vi "HEWH Inlet Outlet Temperature Average.vi"(0 "Remove 15 Seconds Input":T2 {"Hot Water Total (Gal)" format="%#.6f"; "Software Elapsed Time (s)" format="%#.6f"; "Cold Water Total (Gal)" format="%#.6f"}, 1 "Test Type":T1, 11 "error in (no error)":errorcluster) -> (4 "Remove 15 Seconds Output":T2 {"Hot Water Total (Gal)" format="%#.6f"; "Software Elapsed Time (s)" format="%#.6f"; "Cold Water Total (Gal)" format="%#.6f"}, 14 "Time_15s":dbl, 15 "error out":errorcluster)   [LabVIEW 2023]
uses:
  Type Definitions/HEWH Remove 15 Seconds.ctl
  Type Definitions/HEWH Test Type.ctl
panel:
  out "Array":dbl[][](array[numeric])
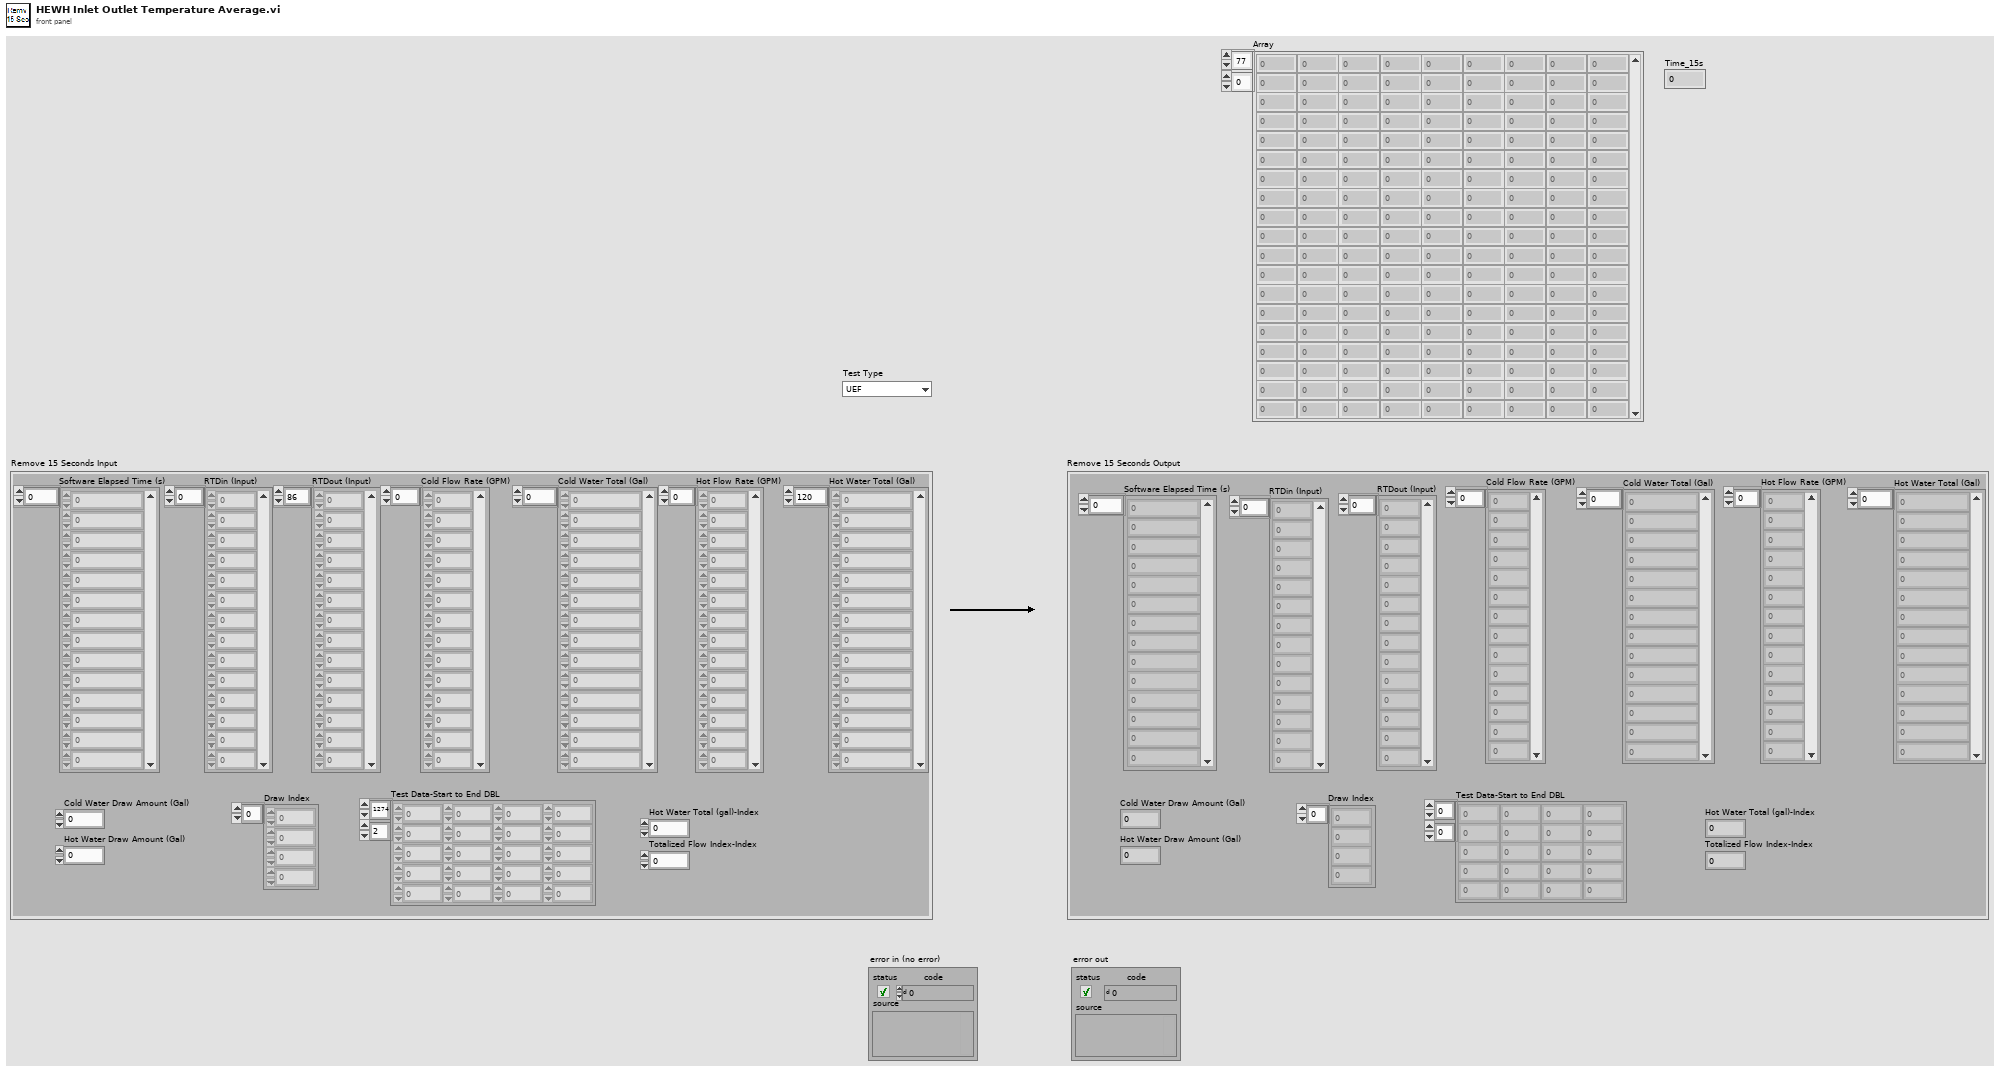
[diagram p1: front panel]
types:
  T1 = typedef "HEWH Test Type.ctl" = enum16{"UEF", "FHD"}
  T2 = typedef "HEWH Remove 15 Seconds.ctl" = cluster{"Cold Water Total (Gal)":dbl[], "Software Elapsed Time (s)":dbl[], "RTDin (Input)":dbl[], "RTDout (Input)":dbl[], "Cold Flow Rate (GPM)":dbl[], "Hot Flow Rate (GPM)":dbl[], "Hot Water Total (Gal)":dbl[], "Cold Water Draw Amount (Gal)":dbl, "Hot Water Draw Amount (Gal)":dbl, "Draw Index":i32[], "Test Data-Start to End DBL":dbl[][], "Hot Water Total (gal)-Index":i32, "Totalized Flow Index-Index":i32}
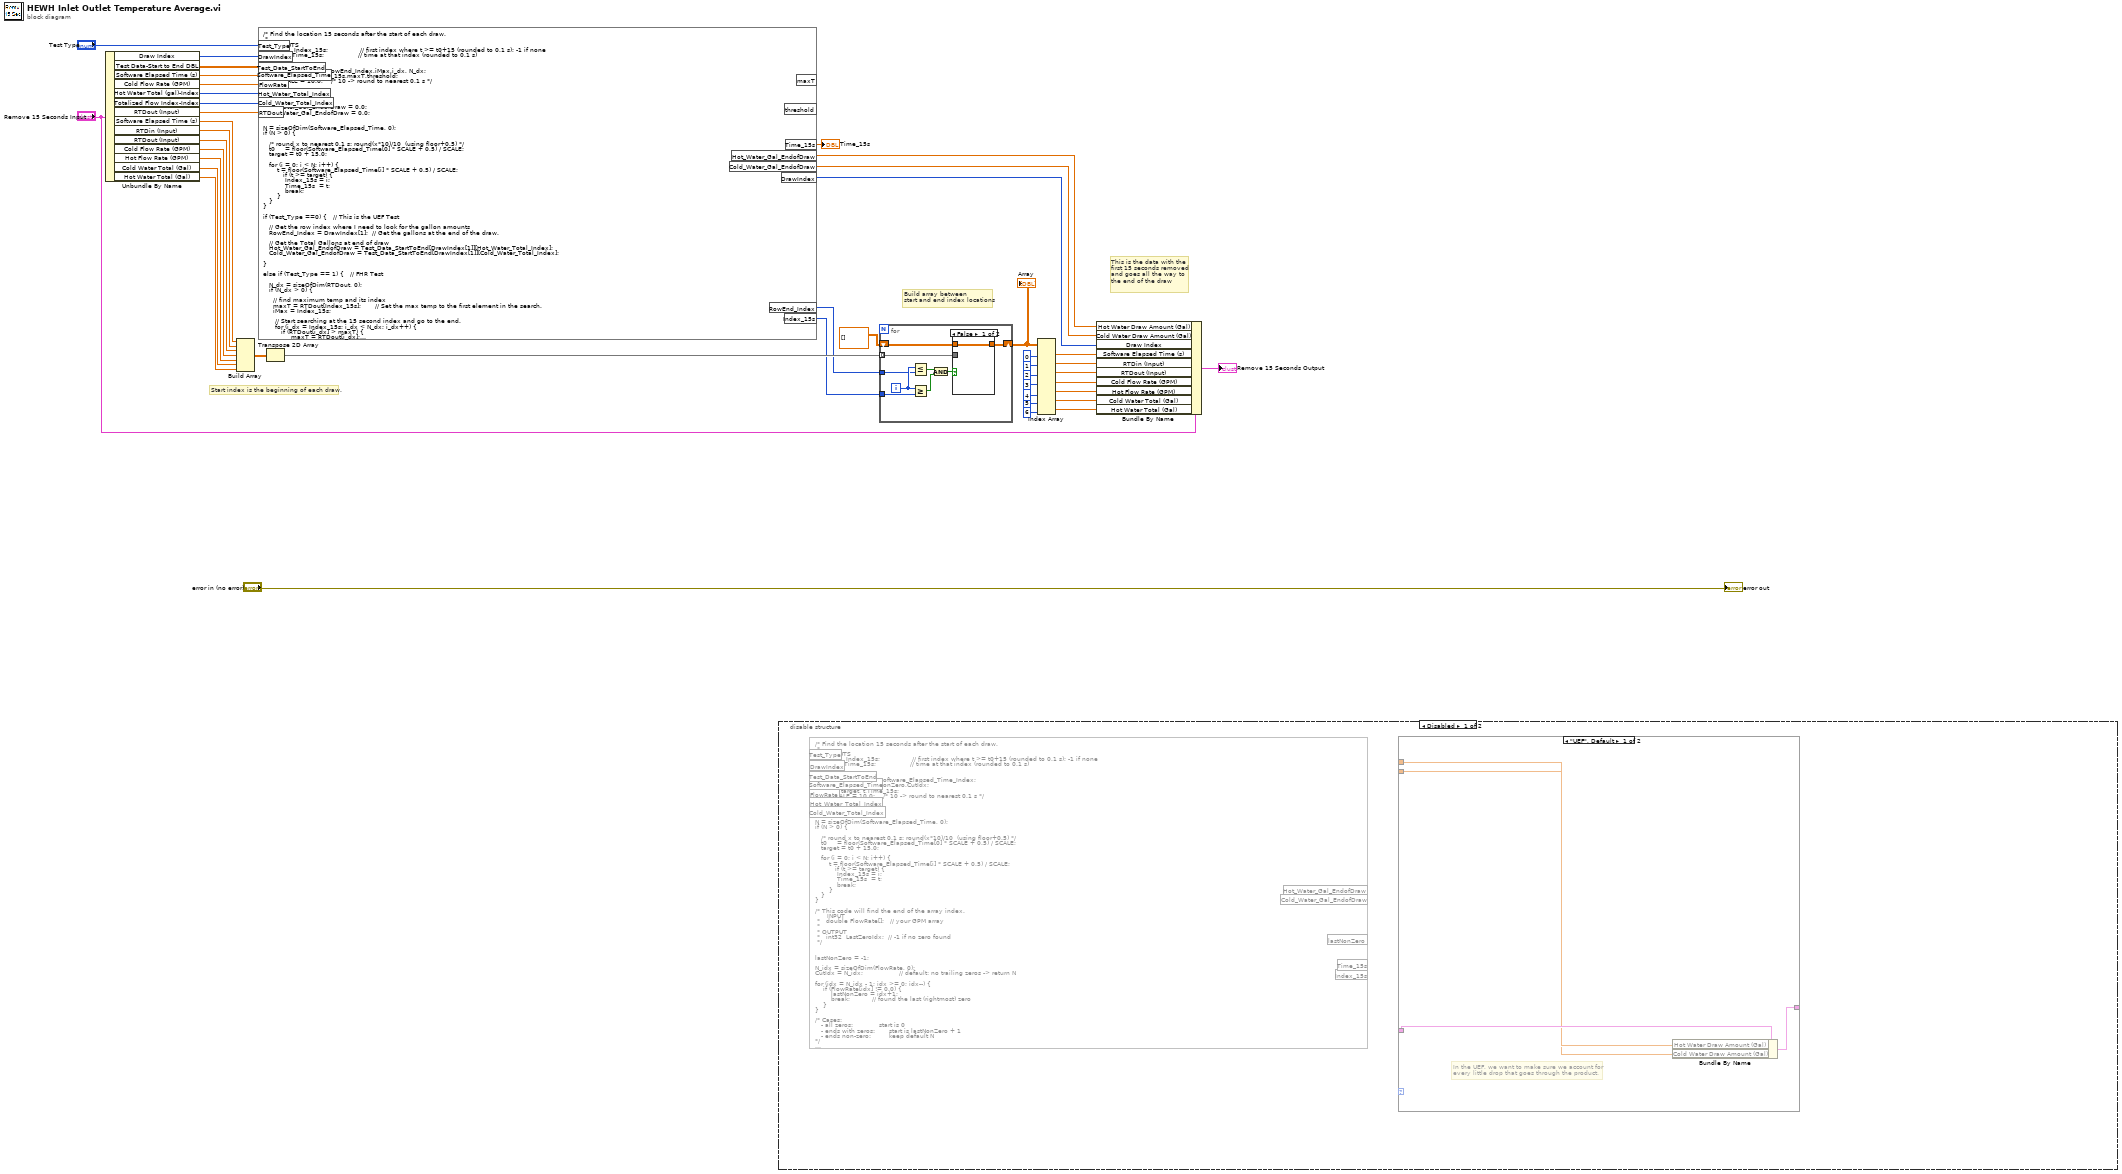
[diagram p0: block diagram]
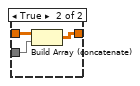
[diagram p2: hidden frame]
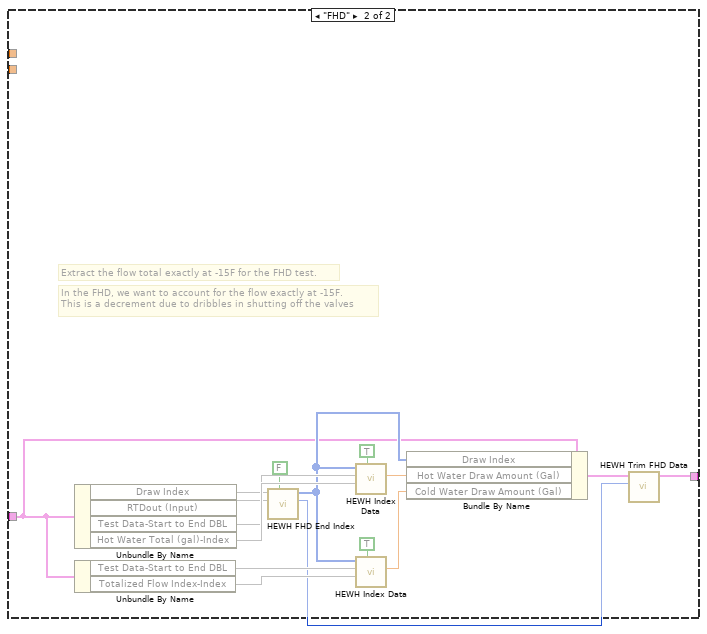
[diagram p3: hidden frame]
diagram:
  # "Start index is the beginning of each draw."
  # "Build array between\nstart and end index locations"
  # "This is the data with the\nfirst 15 seconds removed\nand goes all the way to\nthe end of the draw"
  n1 = Unbundle By Name("Remove 15 Seconds Input") -> ("Draw Index"=w23:i32[], "Test Data-Start to End DBL"=w22:dbl[][], "Software Elapsed Time (s)"=w32:dbl[], "Cold Flow Rate (GPM)"=w33:dbl[], "Hot Water Total (gal)-Index"=w20:i32, "Totalized Flow Index-Index"=w19:i32, "RTDout (Input)"=w18:dbl[], "Software Elapsed Time (s)"=w35:dbl[], "RTDin (Input)"=w40:dbl[], "RTDout (Input)"=w39:dbl[], "Cold Flow Rate (GPM)"=w38:dbl[], "Hot Flow Rate (GPM)"=w37:dbl[], "Cold Water Total (Gal)"=w36:dbl[], "Hot Water Total (Gal)"=w34:dbl[])
  n2 = Build Array(w35, w40, w39, w38, w37, w36, w34) -> (w41:dbl[][])
  n3 = formula code="/* Find the location 15 seconds after the start of each draw. \n *\n * OUTPUTS\n *   int32  Index_15s;                // first index where t >= t0+15 (rounded to 0.1 s); -1 if none\n *   float  Time_15s;                 // time at that index (rounded to 0.1 s)\n */\n\nint32 i, N,Index_15s,RowEnd_Index,iMax,i_dx, N_dx;\nfloat t0, target, t,Time_15s,maxT,threshold;\nfloat SCALE = 10.0;    /* 10 -> round to nearest 0.1 s */\n\nIndex_15s = -1;\nTime_15s  = 0.0;\nRowEnd_Index = -1;\nHot_Water_Gal_EndofDraw = 0.0;\nCold_Water_Gal_EndofDraw = 0.0;\n\n\nN = sizeOfDim(Software_Elapsed_Time, 0);\nif (N > 0) {\n\n   /* round x to nearest 0.1 s: round(x*10)/10  (using floor+0.5) */\n   t0     = floor(Software_Elapsed_Time[0] * SCALE + 0.5) / SCALE;\n   target = t0 + 15.0;\n\n   for (i = 0; i < N; i++) {\n       t = floor(Software_Elapsed_Time[i] * SCALE + 0.5) / SCALE;\n          if (t >= target) {\n           Index_15s = i;\n           Time_15s  = t;\n           break;\n       }\n   }\n}\n\nif (Test_Type ==0) {   // This is the UEF Test\n\n   // Get the row index where I need to look for the gallon amounts\n   RowEnd_Index = DrawIndex[1];  // Get the gallons at the end of the draw.\n\n   // Get the Total Gallons at end of draw\n   Hot_Water_Gal_EndofDraw = Test_Data_StartToEnd[DrawIndex[1]][Hot_Water_Total_Index];\n   Cold_Water_Gal_EndofDraw = Test_Data_StartToEnd[DrawIndex[1]][Cold_Water_Total_Index];\n\n}\n\nelse if (Test_Type == 1) {   // FHR Test\n\n   N_dx = sizeOfDim(RTDout, 0);\n   if (N_dx > 0) {\n     \n     // find maximum temp and its index\n     maxT = RTDout[Index_15s];       // Set the max temp to the first element in the search.\n     iMax = Index_15s;\n\n      // Start searching at the 15 second index and go to the end.\n      for (i_dx = Index_15s; i_dx < N_dx; i_dx++) {\n         if (RTDout[i_dx] > maxT) { \n              maxT = RTDout[i_dx];\n              iMax = i_dx;\n         }\n      }\n\n      // threshold at max - 15°F\n      threshold = maxT - 15.0;\n      \n      // reset for this branch\n      RowEnd_Index = -1;\n\n      // *** scan forward from the maximum index ***\n      for (i_dx = iMax; i_dx <= N_dx; i_dx++) {\n          if (RTDout[i_dx] <= threshold) {\n            RowEnd_Index = i_dx;   // first point = (maxT - 15)\n            break;\n         }\n      }\n\n       // Get the absolute array position for Draw Index (this is the end position)\n       DrawIndex[1] = DrawIndex[0] + RowEnd_Index;   /* absolute end-of-draw position */ \n\n      // grab gallons at that index if found\n      if (RowEnd_Index >= 0 && RowEnd_Index < sizeOfDim(Test_Data_StartToEnd, 0)) {\n         Hot_Water_Gal_EndofDraw  = Test_Data_StartToEnd[DrawIndex[1]][Hot_Water_Total_Index];;\n         Cold_Water_Gal_EndofDraw = Test_Data_StartToEnd[DrawIndex[1]][Cold_Water_Total_Index];\n      }\n   }\n}"("FlowRate"=w33, "Software_Elapsed_Time"=w32, "DrawIndex"=w23, "Test_Data_StartToEnd"=w22, "Test_Type"="Test Type", "Hot_Water_Total_Index"=w20, "Cold_Water_Total_Index"=w19, "RTDout"=w18) -> ("RowEnd_Index"=w13:i32, "Index_15s"=w14:i32, "Time_15s"=→"Time_15s":dbl, "Hot_Water_Gal_EndofDraw"=w4:dbl, "Cold_Water_Gal_EndofDraw"=w3:dbl, "DrawIndex"=w5:i32[])  [unwired: 2 out]
  n4 = Transpose 2D Array(2D array=w41) -> (transposed array=w17:dbl[][])
  n5 = disable-structure shown="Disabled" {
    frame Disabled {
      n6 = formula code="/* Find the location 15 seconds after the start of each draw. \n *\n * OUTPUTS\n *   int32  Index_15s;                // first index where t >= t0+15 (rounded to 0.1 s); -1 if none\n *   float  Time_15s;                 // time at that index (rounded to 0.1 s)\n */\n\nint32 i, N,Index_15s,Software_Elapsed_Time_Index;\nint32 idx, N_idx, lastNonZero,CutIdx;\nfloat t0, target, t,Time_15s;\nfloat SCALE = 10.0;    /* 10 -> round to nearest 0.1 s */\n\nIndex_15s = -1;\nTime_15s  = 0.0;\n\nN = sizeOfDim(Software_Elapsed_Time, 0);\nif (N > 0) {\n\n   /* round x to nearest 0.1 s: round(x*10)/10  (using floor+0.5) */\n   t0     = floor(Software_Elapsed_Time[0] * SCALE + 0.5) / SCALE;\n   target = t0 + 15.0;\n\n   for (i = 0; i < N; i++) {\n       t = floor(Software_Elapsed_Time[i] * SCALE + 0.5) / SCALE;\n          if (t >= target) {\n           Index_15s = i;\n           Time_15s  = t;\n           break;\n       }\n   }\n}\n\n/* This code will find the end of the array index.  \n      INPUT\n *   double FlowRate[];   // your GPM array\n *\n * OUTPUT\n *   int32  LastZeroIdx;  // -1 if no zero found\n */\n\n\nlastNonZero = -1;\n\nN_idx = sizeOfDim(FlowRate, 0);\nCutIdx = N_idx;                  // default: no trailing zeros -> return N\n\nfor (idx = N_idx - 1; idx >= 0; idx--) {\n    if (FlowRate[idx] != 0.0) {\n        lastNonZero = idx+1;\n        break;           // found the last (rightmost) zero\n    }\n}\n\n/* Cases:\n   - all zeros:             start is 0\n   - ends with zeros:       start is lastNonZero + 1\n   - ends non-zero:         keep default N\n*/\n\nif (lastNonZero == -1) {\n    CutIdx = 0;                 // e.g., [0,0,0] -> 0\n} \nelse if (lastNonZero < N_idx - 1) {\n    CutIdx = lastNonZero+1;   // e.g., [20,0,0,0] -> 1\n}\n/* else leave CutIdx = N (e.g., [1,2,3] -> 3) */\n\n// This section of code finds the hot and cold water totalized gallons\n\nif (Test_Type ==0) {   // This is the UEF Test\n\n// Get the row index where I need to look for the gallon amounts\nSoftware_Elapsed_Time_Index = DrawIndex[1];\n\n// Get the Total Gallons\nHot_Water_Gal_EndofDraw = Test_Data_StartToEnd[Software_Elapsed_Time_Index][Hot_Water_Total_Index];\nCold_Water_Gal_EndofDraw = Test_Data_StartToEnd[Software_Elapsed_Time_Index][Cold_Water_Total_Index];\n\n}\n\n// In this section, I need to look for -15F decrement exactly and get that location.\n// So, look at the RTDout, find the maximum temperature in the draw, then subtract 15 degrees, then move \n// your index backward until you get a 15 degree decrement, this is your new stop index. This is index location is\n// your new \"lastNonZero\" index location. then go ahead and grab the \"Hot_Water_Gal_EndofDraw\" and\n// \"Cold_Water_Gal_EndofDraw\""() -> ()  [unwired: 7 in, 5 out]
      n7 = case shown="\"UEF\", Default" {
        selector: _ -> [_ _]
        tunnel: _ -> [w45 w47]
        tunnel: [w46 w49] -> _
        tunnel: _ -> [w44 _]
        tunnel: _ -> [w43 _]
        frame "UEF", Default {
          # "In the UEF, we want to make sure we account for\nevery little drop that goes through the product."
          n8 = Bundle By Name(cluster=w45, "Hot Water Draw Amount (Gal)"=w44, "Cold Water Draw Amount (Gal)"=w43) -> (w46:cluster{})
        }
        frame "FHD" {
          # "In the FHD, we want to account for the flow exactly at -15F.\nThis is a decrement due to dribbles in shutting off the valves"
          # "Extract the flow total exactly at -15F for the FHD test."
          n9 = Unbundle By Name(w47) -> ("Draw Index"=w57, "RTDout (Input)"=w56, "Test Data-Start to End DBL"=w55, "Hot Water Total (gal)-Index"=w61)
          n10 = Unbundle By Name(w47) -> ("Test Data-Start to End DBL"=w59, "Totalized Flow Index-Index"=w60)
          n11 = call "HEWH FHD End Index.vi"("Fixed Search?"=FALSE, "RTDout"=w56, "Draw Index"=w57) -> ("Decrement Amount"=w51:i32, "Updated FHD End Index"=w54:i32[])  [unwired: 6 in, 1 out]
          n12 = call "HEWH Index Data.vi"("Basic Index?"=TRUE, "Data Index Location"=w61, "Test Data-Start to End DBL"=w55, "Draw Index"=w54) -> ("Basic Index Output"=w53:dbl)  [unwired: 5 in, 2 out]
          n13 = call "HEWH Index Data.vi"("Basic Index?"=TRUE, "Data Index Location"=w60, "Test Data-Start to End DBL"=w59, "Draw Index"=w54) -> ("Basic Index Output"=w52:dbl)  [unwired: 5 in, 2 out]
          n14 = Bundle By Name(cluster=w47, "Draw Index"=w54, "Hot Water Draw Amount (Gal)"=w53, "Cold Water Draw Amount (Gal)"=w52) -> (w50:cluster{})
          n15 = call "HEWH Trim FHD Data.vi"("Decrement Amount"=w51, "Remove 15 Seconds Input in"=w50) -> ("Remove 15 Seconds Input out"=w49:T2)  [unwired: 8 in, 1 out]
        }
      }
    }
    frame Enabled {
    }
  }
  n16 = for {
    tunnel: w17 -> [w71] mode=indexing
    shift-right: [w69] -> w15
    shift-left: dbl[][] [] -> [w70]
    tunnel: w13 -> [w66]
    tunnel: w14 -> [w68]
    i -> [w67]
    n17 = Less Or Equal?(x=w67, y=w66) -> (x <= y?=w65:bool)
    n18 = Greater Or Equal?(x=w67, y=w68) -> (x >= y?=w64:bool)
    n19 = And(x=w65, y=w64) -> (x .and. y?=w63:bool)
    n20 = case shown="False" w63 {
      tunnel: w71 -> [_ w75]
      tunnel: w70 -> [w72 w74]
      tunnel: [w72 w73] -> w69
      frame False {
      }
      frame True {
        n21 = Build Array (concatenate)(w74, w75) -> (w73:dbl[][])
      }
    }
  }
  "Array" <- w15
  n22 = Index Array(array=w15, index (col) #1=0 ("disabled index (col)"), index (col) #2=1 ("index (col)"), index (col) #3=2 ("index (col)"), index (col) #4=3 ("index (col)"), index (col) #5=4 ("index (col)"), index (col) #6=5 ("index (col)"), index (col) #7=6 ("index (col)")) -> (element #1=w12:dbl[], element #2=w11:dbl[], element #3=w10:dbl[], element #4=w9:dbl[], element #5=w8:dbl[], element #6=w7:dbl[], element #7=w6:dbl[])  [unwired: 7 in]
  n23 = Bundle By Name(cluster="Remove 15 Seconds Input", "Hot Water Draw Amount (Gal)"=w4, "Cold Water Draw Amount (Gal)"=w3, "Draw Index"=w5, "Software Elapsed Time (s)"=w12, "RTDin (Input)"=w11, "RTDout (Input)"=w10, "Cold Flow Rate (GPM)"=w9, "Hot Flow Rate (GPM)"=w8, "Cold Water Total (Gal)"=w7, "Hot Water Total (Gal)"=w6) -> (→"Remove 15 Seconds Output":T2)
  "error out" <- "error in (no error)"
